vi "Is Window Foreground.vi"(8 "error in (no error)":errorcluster, 11 "hWnd":i32) -> (0 "error out":errorcluster, 2 "Is Foreground?":bool)   [LabVIEW 2020, in "PicoG-Processor.lvlib"]
uses:
  PicoG-Processor.lvlib
  user32.dll
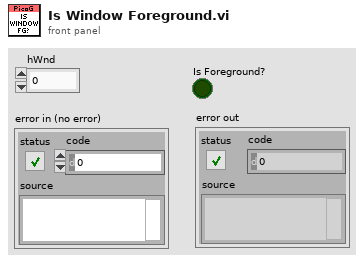
[diagram p1: front panel]
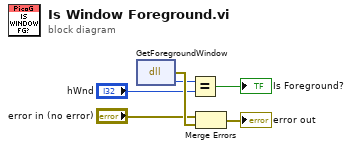
[diagram p0: block diagram]
diagram:
  n1 = dll-call lib="user32.dll" fn="GetForegroundWindow"() -> (error out=w6:errorcluster, "return type"=w1:i32)  [unwired: 3 in, 1 out]
  n2 = Equal?(x=w1, y="hWnd") -> (x = y?=→"Is Foreground?":bool)
  n3 = Merge Errors("error in (no error)", w6) -> (→"error out":errorcluster)
